vi "takesampleBK.vi"(8 "error in (no error)":errorcluster, 11 "VISA resource name":refnum<visa-resource-name>) -> (0 "error out":errorcluster, 2 "current sample":string, 3 "VISA resource name out":refnum<visa-resource-name>)   [LabVIEW 2021]
panel:
  out "return count":u32
  out "time (s)":dbl
  in  "Filename":path=path "data/test.lvm"
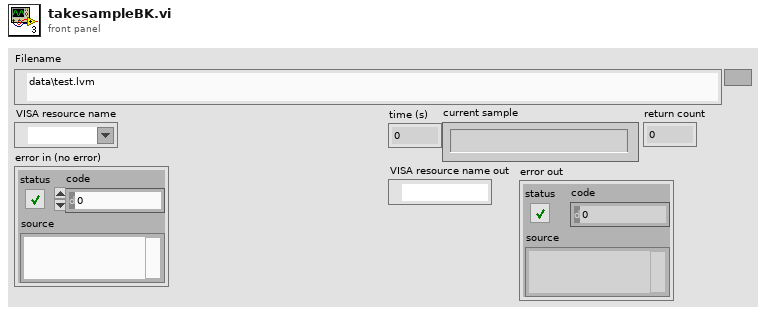
[diagram p1: front panel]
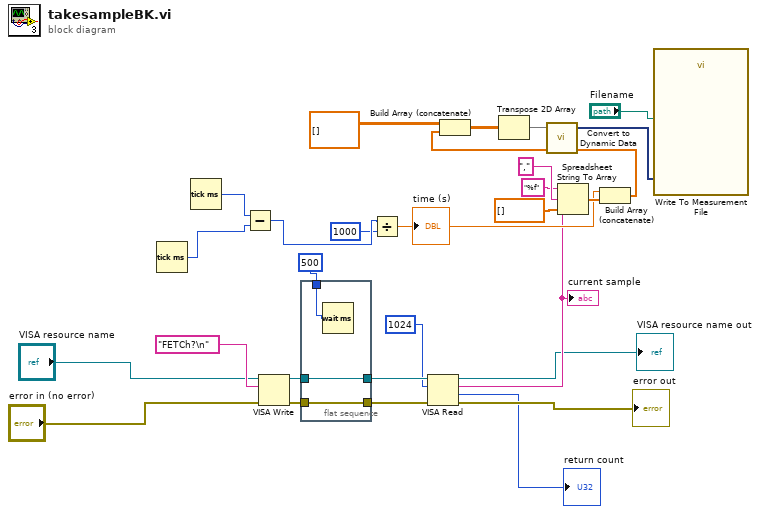
[diagram p0: block diagram]
diagram:
  n1 = Tick Count (ms)() -> (millisecond timer value=w28:u32)
  n2 = Tick Count (ms)() -> (millisecond timer value=w15:u32)
  n3 = Subtract(x=w15, y=w28) -> (x-y=w14:u32)
  n4 = VISA Write(VISA resource name="VISA resource name", write buffer="FETCh?\n" ("Command"), error in (no error)="error in (no error)") -> (VISA resource name out=w20:refnum<visa-resource-name>, error out=w22:errorcluster)  [unwired: 1 out]
  n5 = flat-sequence {
    tunnel: w22 -> [w31]
    tunnel: [w31] -> w21
    tunnel: w20 -> [w30]
    tunnel: [w30] -> w19
    tunnel: u32 500 ("delay before read (ms)") -> [w29]
    frame #0 {
      n6 = Wait (ms)(milliseconds to wait=w29) -> ()  [unwired: 1 out]
    }
  }
  n7 = Divide(x=w14, y=u32 1000) -> (x/y=w8:dbl)
  "time (s)" <- w8
  n8 = VISA Read(VISA resource name=w19, byte count=u32 1024, error in (no error)=w21) -> (VISA resource name out=→"VISA resource name out":refnum<visa-resource-name>, read buffer=w6:string, return count=→"return count":u32, error out=→"error out":errorcluster)
  "current sample" <- w6
  n9 = Spreadsheet String To Array(delimiter (Tab)=",", format string="%f", spreadsheet string=w6, array type (2D Dbl)=dbl[] []) -> (array=w9:dbl[])
  n10 = Build Array (concatenate)(w8, w9) -> (w7:dbl[])
  n11 = Build Array (concatenate)(dbl[][] [], w7) -> (w23:dbl[][])
  n12 = Transpose 2D Array(2D array=w23) -> (transposed array=w24:dbl[][])
  n13 = call "Convert to Dynamic Data"("2D Array"=w24) -> ("Dynamic Data Type"=w26:dynamicdata)  [unwired: 3 in]
  n14 = call "Write To Measurement File"("Signals"=w26, "Filename"="Filename") -> ()  [unwired: 15 in, 3 out]
